vi "STL- STLToArray.vi"(8 "Boolean":bool, 10 "String":string, 11 "file (use dialog)":path) -> (2 "Array 3":dbl[][](array[numeric]))   [LabVIEW 2019]
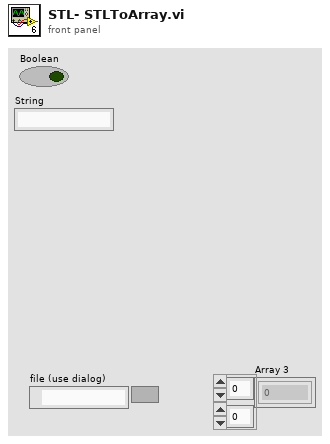
[diagram p1: front panel]
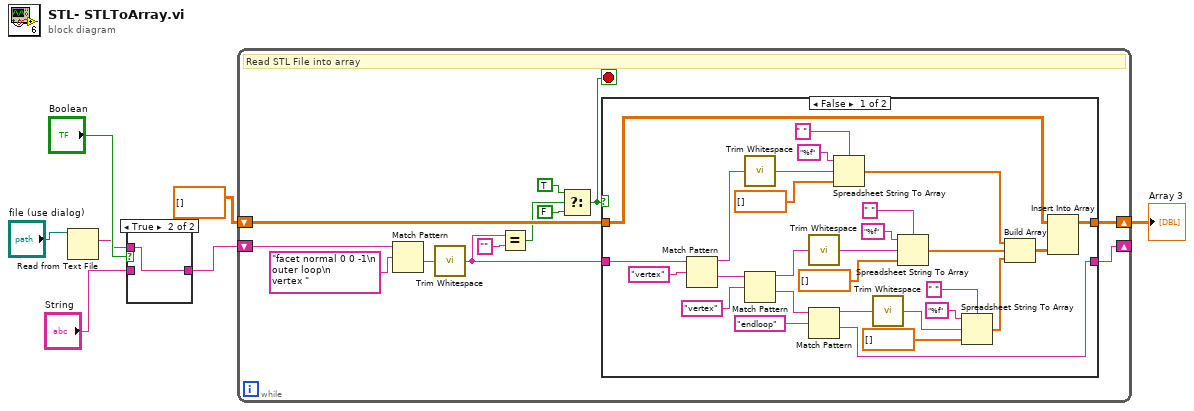
[diagram p0: block diagram]
diagram:
  n1 = Read from Text File(file (use dialog)="file (use dialog)") -> (text=w2:string)  [unwired: 3 in, 3 out]
  n2 = case shown="True" "Boolean" {
    tunnel: "String" -> [w8 _]
    tunnel: w2 -> [_ w9]
    tunnel: [w8 w9] -> w1
    frame False {
    }
    frame True {
    }
  }
  n3 = while {
    shift-right: [w11] -> _
    shift-left: w1 -> [w19]
    shift-right: [w17] -> w7
    shift-left: dbl[][] [] ("Array 3") -> [w18]
    stop <- w10 stop-if-true
    # "Read STL File into array"
    n4 = Match Pattern(string=w19, regular expression="facet normal 0 0 -1\n    outer loop\n      vertex ") -> (after substring=w20:string)  [unwired: 1 in, 3 out]
    n5 = call <vilib>:"Trim Whitespace.vi"("string"=w20) -> ("trimmed string"=w16:string)  [unwired: 1 in]
    n6 = Equal?(x=w16, y="") -> (x = y?=w14:bool)
    n7 = Select(t=TRUE, s=w14, f=FALSE) -> (s? t:f=w10:bool)
    n8 = case shown="False" w10 {
      tunnel: w18 -> [w48 w50]
      tunnel: [w47 w50] -> w17
      tunnel: w16 -> [w46 w51]
      tunnel: [w23 w51] -> w11
      frame False {
        n9 = Match Pattern(string=w46, regular expression="vertex") -> (before substring=w41:string, after substring=w33:string)  [unwired: 1 in, 2 out]
        n10 = call <vilib>:"Trim Whitespace.vi"("string"=w41) -> ("trimmed string"=w40:string)  [unwired: 1 in]
        n11 = Match Pattern(string=w33, regular expression="vertex") -> (before substring=w35:string, after substring=w24:string)  [unwired: 1 in, 2 out]
        n12 = call <vilib>:"Trim Whitespace.vi"("string"=w35) -> ("trimmed string"=w34:string)  [unwired: 1 in]
        n13 = Match Pattern(string=w24, regular expression="endloop") -> (before substring=w26:string, after substring=w23:string)  [unwired: 1 in, 2 out]
        n14 = Spreadsheet String To Array(delimiter (Tab)=" ", format string="%f", spreadsheet string=w40, array type (2D Dbl)=dbl[] []) -> (array=w32:dbl[])
        n15 = call <vilib>:"Trim Whitespace.vi"("string"=w26) -> ("trimmed string"=w25:string)  [unwired: 1 in]
        n16 = Spreadsheet String To Array(delimiter (Tab)=" ", format string="%f", spreadsheet string=w34, array type (2D Dbl)=dbl[] []) -> (array=w31:dbl[])
        n17 = Spreadsheet String To Array(delimiter (Tab)=" ", format string="%f", spreadsheet string=w25, array type (2D Dbl)=dbl[] []) -> (array=w22:dbl[])
        n18 = Build Array(w32, w31, w22) -> (w49:dbl[][])
        n19 = Insert Into Array(array=w48, new element=w49) -> (w47:dbl[][])  [unwired: 2 in]
      }
      frame True {
      }
    }
  }
  "Array 3" <- w7
